vi "Element Contents.vi"(10 "Name":string, 11 "XML in":string) -> (2 "Content":string, 3 "XML Out":string)   [LabVIEW 2019]
doc: "This VI is Developed by Anish Prabu T.\n\nCopyright © 2006, email:anishprabu243@yahoo.co.in.\nAll rights reserved."
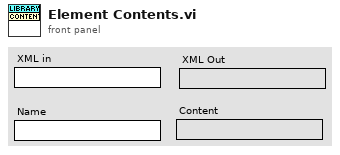
[diagram p1: front panel]
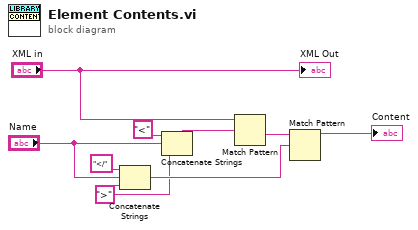
[diagram p0: block diagram]
diagram:
  w1 = ">" ("Substring")
  n1 = Concatenate Strings("</" ("Substring"), "Name", w1) -> (w5:string)
  n2 = Concatenate Strings("<" ("Substring"), "Name", w1) -> (w2:string)
  n3 = Match Pattern(string="XML in", regular expression=w2) -> (after substring=w8:string)  [unwired: 1 in, 3 out]
  n4 = Match Pattern(string=w8, regular expression=w5) -> (before substring=→"Content":string)  [unwired: 1 in, 3 out]
  "XML Out" <- "XML in"
